vi "RadioOpTester.vi"() -> ()   [LabVIEW 2016]
uses:
  <vilib>/Instr/_visa.llb/VISA Configure Serial Port (Instr).vi
panel:
  out "bytes":u32
  out "read buffer":string
  out "available?":bool
  in  "VISA resource name":refnum<visa-resource-name>
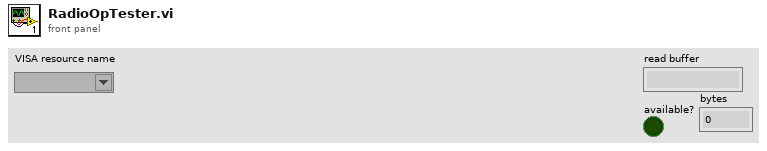
[diagram p1: front panel]
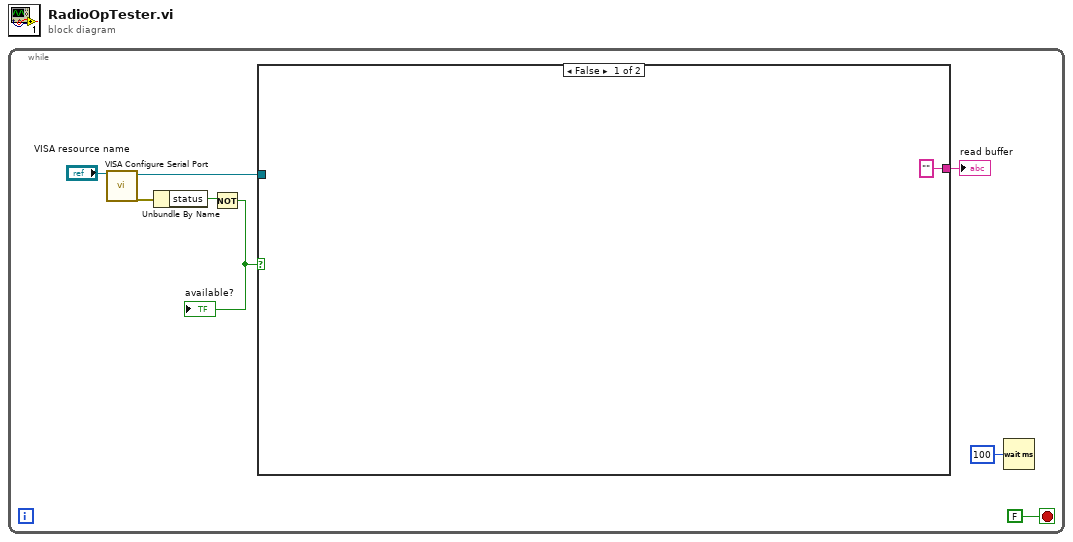
[diagram p0: block diagram]
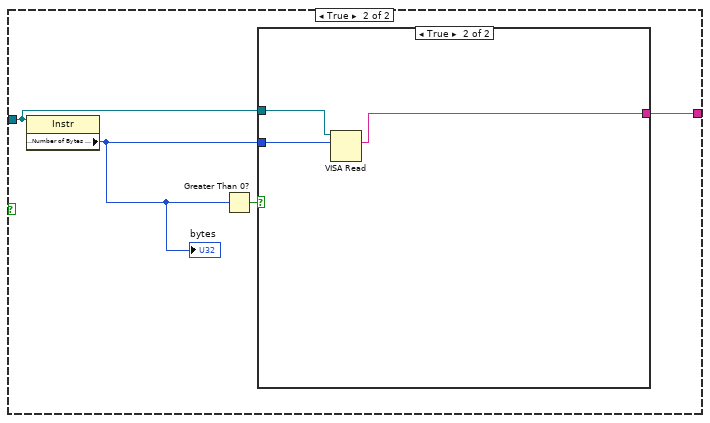
[diagram p2: hidden frame]
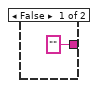
[diagram p3: hidden frame]
diagram:
  n1 = while {
    stop <- FALSE stop-if-true
    n2 = call-poly "VISA Configure Serial Port"("VISA resource name"="VISA resource name") -> ("VISA resource name out"=w5:refnum<visa-resource-name>, "error out"=w4:errorcluster)  [unwired: 13 in]
    n3 = Unbundle By Name(w4) -> ("status"=w3:bool)
    n4 = Not(x=w3) -> (.not. x?=w2:bool)
    "available?" <- w2
    n5 = case shown="False" w2 {
      tunnel: w5 -> [_ w11]
      tunnel: ["" ("read buffer") w10] -> w1
      frame False {
      }
      frame True {
        n6 = property class="Instr"(reference=w11) -> ("Serial Settings:Number of Bytes at Serial Port"=w12:u32)  [unwired: 1 in, 2 out]
        "bytes" <- w12
        n7 = Greater Than 0?(x=w12) -> (x > 0?=w13:bool)
        n8 = case shown="True" w13 {
          tunnel: w12 -> [_ w16]
          tunnel: w11 -> [_ w17]
          tunnel: ["" ("read buffer") w15] -> w10
          frame False {
          }
          frame True {
            n9 = VISA Read(VISA resource name=w17, byte count=w16) -> (read buffer=w15:string)  [unwired: 1 in, 3 out]
          }
        }
      }
    }
    "read buffer" <- w1
    n10 = Wait (ms)(milliseconds to wait=u32 100) -> ()  [unwired: 1 out]
  }
